vi "ReadCsvControlSpreadsheet.vi"(0 "Robot ID":string="984", 1 "Motor ID":string="Drive Left Center") -> (2 "Can Bus ID":string, 3 "PWM Channel":string, 4 "PDP Channel ID":string)   [LabVIEW 2017]
uses:
  <vilib>/Utility/file.llb/Read Delimited Spreadsheet (string).vi
panel:
  in  "file path for Win":path=path "C:/git/981LabViewComponents/ControlSpreadsheet.csv"
  in  "file path for linux":path=path "/home/lvuser/ControlSpreadsheet.csv"
  out "Row with Info":i32
  out "Motor ID from Row x":string
  out "Number of Rows":i32
  out "Robot ID from Row x":string
  out "Number of Columns":i32
  out "subarray":string[](array[string])
  out "all rows":string[][](array[string])
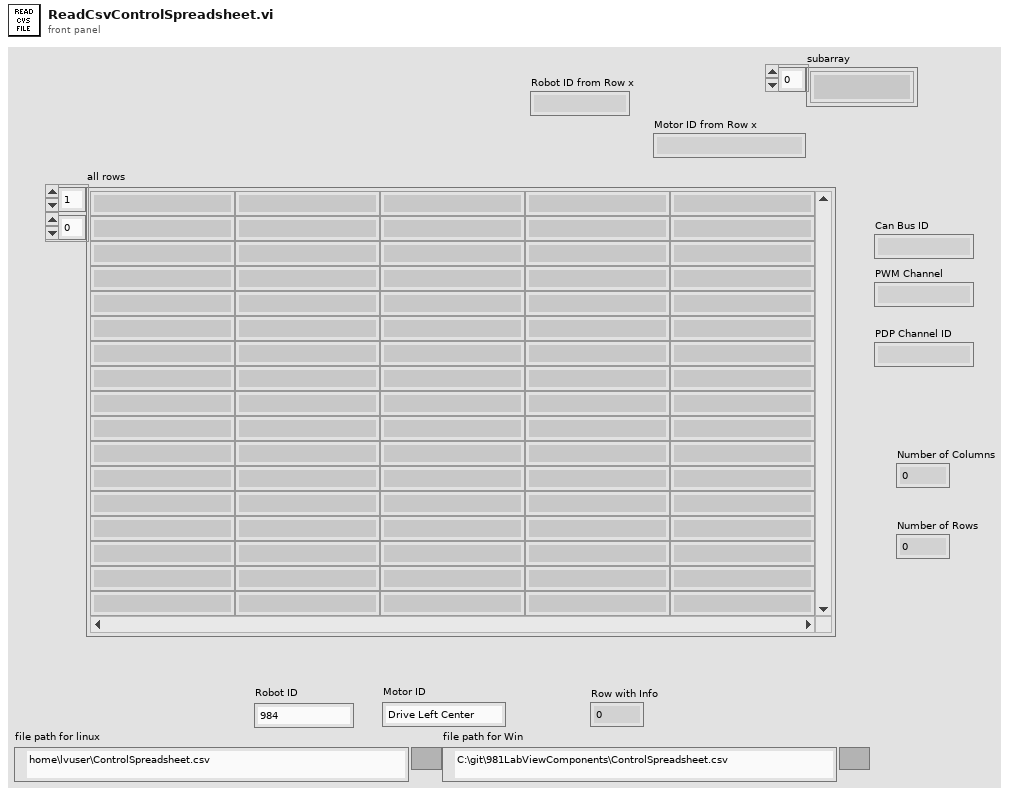
[diagram p1: front panel]
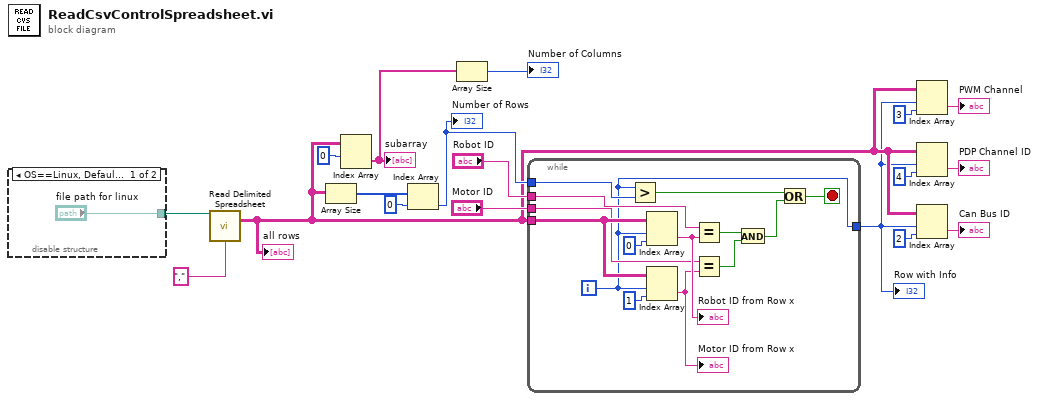
[diagram p0: block diagram]
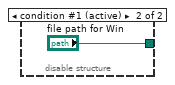
[diagram p2: hidden frame]
diagram:
  n1 = disable-structure shown="OS==Linux, Default" {
    disable-tunnel: ["file path for linux" "file path for Win"] -> w1
    frame condition #0 {
    }
    frame condition #1 (active) {
    }
  }
  n2 = call-poly <vilib>:"Read Delimited Spreadsheet.vi"("file path (dialog if empty)"=w1, "delimiter (\\t)"="," ("delimiter (\\t)")) -> ("all rows"=w9:string[][])  [unwired: 8 in, 5 out]
  "all rows" <- w9
  n3 = Array Size(array=w9) -> (size(s)=w14:i32[])
  n4 = Index Array(array=w9, index (row)=0) -> (element=w16:string[])  [unwired: 1 in]
  "subarray" <- w16
  n5 = Index Array(array=w14, index=0) -> (element=w12:i32)
  "Number of Rows" <- w12
  n6 = Array Size(array=w16) -> (size(s)=→"Number of Columns":i32)
  n7 = while {
    tunnel: w9 -> [w27]
    tunnel: w12 -> [w32]
    tunnel: "Robot ID" -> [w29]
    tunnel: "Motor ID" -> [w25]
    tunnel: [w21] -> w8
    i -> [w21]
    stop <- w31 stop-if-true
    n8 = Greater?(x=w21, y=w32) -> (0:w33:bool)
    n9 = Index Array(array=w27, index (row)=w21, index (col)=0 ("disabled index (col)")) -> (element=w30:string)
    "Robot ID from Row x" <- w30
    n10 = Index Array(array=w27, index (row)=w21, index (col)=1) -> (element=w26:string)
    "Motor ID from Row x" <- w26
    n11 = Equal?(x=w29, y=w30) -> (x = y?=w24:bool)
    n12 = Equal?(x=w25, y=w26) -> (x = y?=w23:bool)
    n13 = And(x=w24, y=w23) -> (x .and. y?=w22:bool)
    n14 = Or(x=w33, y=w22) -> (x .or. y?=w31:bool)
  }
  "Row with Info" <- w8
  n15 = Index Array(array=w9, index (row)=w8, index (col)=3 ("disabled index (col)")) -> (element=→"PWM Channel":string)
  n16 = Index Array(array=w9, index (row)=w8, index (col)=4 ("disabled index (col)")) -> (element=→"PDP Channel ID":string)
  n17 = Index Array(array=w9, index (row)=w8, index (col)=2 ("disabled index (col)")) -> (element=→"Can Bus ID":string)
